vi "SetFileStreamReference.vi"(8 "error in (no error)":errorcluster, 10 "FileStream":refnum<k5>, 11 "connection ID out":T1) -> (0 "error out":errorcluster, 3 "connection ID":T1)   [LabVIEW 2017]
uses:
  <vilib>/addons/InsightCM/MessageBus/TcpApi/controls/TcpMessageReference.ctl
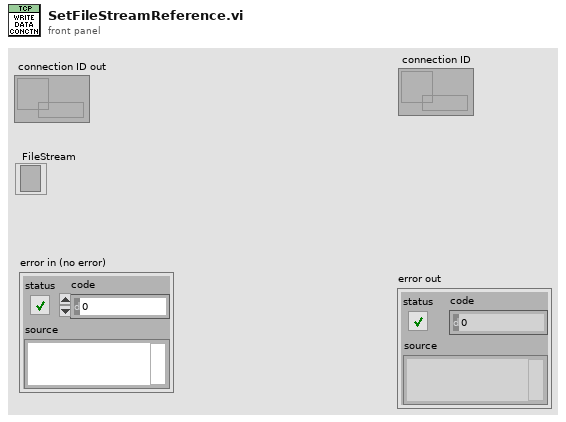
[diagram p1: front panel]
types:
  T1 = typedef "TcpMessageReference.ctl" = refnum<data-value>
  T2 = cluster{"DeviceId":string, "CmdStream":refnum<k5>, "FileStream":refnum<k5>}
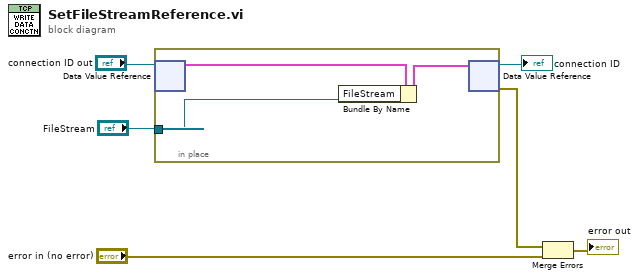
[diagram p0: block diagram]
diagram:
  n1 = in-place {
    in-place-border: "FileStream" -> [w8]
    n2 = in-place-dvr #1("connection ID out") -> (w9:T2)  [unwired: 1 out]
    n3 = Bundle By Name(cluster=w9, "FileStream"=w8) -> (w7:T2)
    n4 = in-place-dvr #1(w7) -> (→"connection ID":T1, w2:errorcluster)
  }
  n5 = Merge Errors(w2, "error in (no error)") -> (→"error out":errorcluster)
